vi "PS_Testing.vi"() -> ()   [LabVIEW 2012]
uses:
  BotSpeakSubs/BotspeakSettingsUsed.vi
  SubVIs/LVPresent_Globals.vi
panel:
  out "Button":bool
  out "Light":u8(slide) scale=0.0..255.0
  in  "LED":cluster{"Red":bool, "Green":bool, "Blue":bool}
  # "Test the ProtoSnap\n\nTry pushing the button or reading the light sensor.  You can click on any of the areas to see the program that is running"
  # "Click these to turn on LEDs!"
  # "Move your finger over the sensor to see the bar change!"
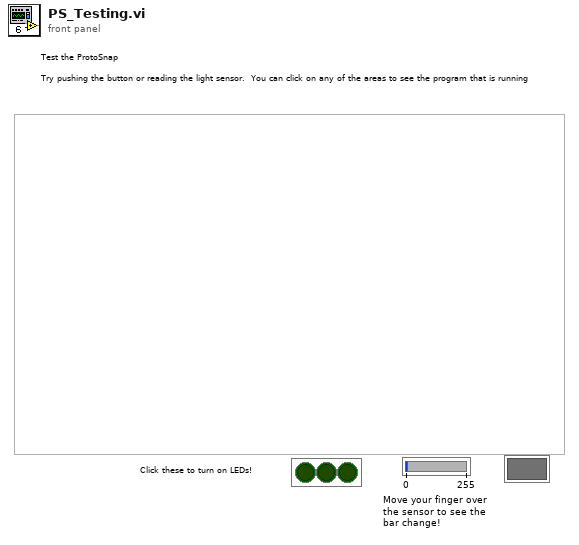
[diagram p1: front panel]
types:
  T1 = typedef "BotSpeak_Control.ctl" = cluster{"Address":string, "Reply EOF":string, "Hardware":string, "Retries":i8, "Timeout":i32}
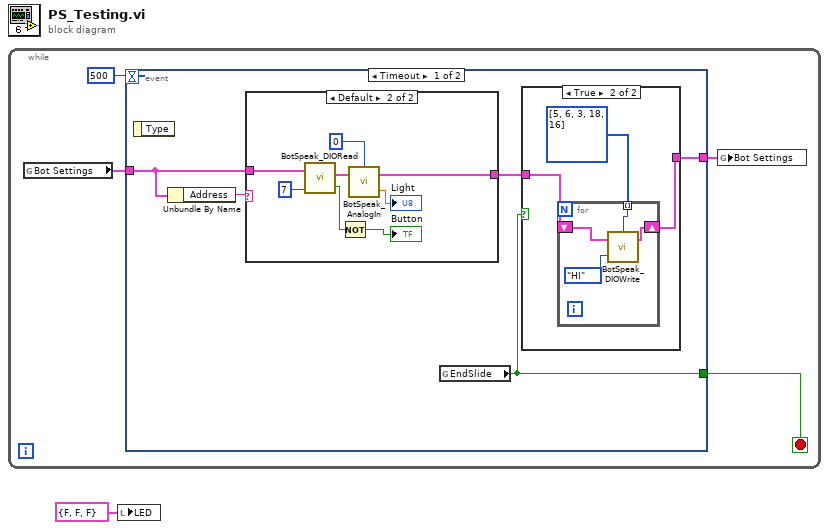
[diagram p0: block diagram]
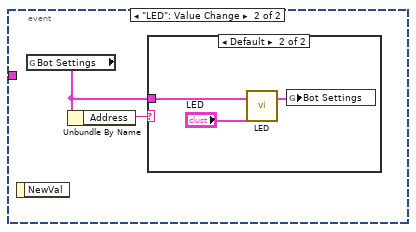
[diagram p4: hidden frame]
diagram:
  n1 = while {
    stop <- w5 stop-if-true
    n2 = global read "BotspeakSettingsUsed.vi" "Bot Settings"() -> (w3:T1)
    n3 = event shown="[0] Timeout" {
      selector: _ -> [_ _]
      dyn-events: _ -> [_ _]
      timeout: 500 -> [_ _]
      tunnel: [w10 _] -> w5
      tunnel: w3 -> [w9 _]
      tunnel: [w6 _] -> w2
      event Timeout {
        n4 = event-data() -> ()  [unwired: 1 in, 1 out]
        n5 = Unbundle By Name(w9) -> ("Address"=w8:string)
        n6 = case shown="Default" w8 {
          tunnel: w9 -> [w19 w21]
          tunnel: [w19 w20] -> w7
          frame "" {
          }
          frame Default {
            n7 = call <userlib>:"BotSpeak_DIORead.vi"("Bot Settings"=w21, "DIO Line"=u32 7) -> ("State"=w24:bool, "Bot Settings out"=w23:T1)  [unwired: 1 in]
            n8 = Not(x=w24) -> (.not. x?=→"Button":bool)
            n9 = call <userlib>:"BotSpeak_AnalogIn.vi"("Bot Settings"=w23, "A/D Channel"=u8 0) -> ("voltage"=→"Light":dbl, "Bot Settings"=w20:T1)  [unwired: 1 in]
          }
        }
        n10 = global read "LVPresent_Globals.vi" "EndSlide"() -> (w10:bool)
        n11 = case shown="True" w10 {
          tunnel: w7 -> [w11 w13]
          tunnel: [w11 w12] -> w6
          frame False {
          }
          frame True {
            n12 = for {
              tunnel: i32[] [5, 6, 3, 18, 16] -> [w18] mode=indexing
              shift-right: [w15] -> w12
              shift-left: w13 -> [w16]
              n13 = call <userlib>:"BotSpeak_DIOWrite.vi"("State"=enum32{"LO", "HI"}."HI", "Bot Settings"=w16, "DIO Line"=w18) -> ("Bot Settings"=w15:T1)  [unwired: 1 out]
            }
          }
        }
      }
      event "LED": Value Change {
        n14 = event-data() -> ()  [unwired: 1 in, 1 out]
        n15 = global read "BotspeakSettingsUsed.vi" "Bot Settings"() -> (w29:T1)
        n16 = Unbundle By Name(w29) -> ("Address"=w28:string)
        n17 = case shown="Default" w28 {
          tunnel: w29 -> [_ w31]
          frame "" {
          }
          frame Default {
            n18 = call "LED.vi"("LED"="LED", "Bot Settings"=w31) -> ("Bot Settings out"=w30:T1)  [unwired: 1 in]
            n19 = global write "BotspeakSettingsUsed.vi" "Bot Settings"(w30) -> ()
          }
        }
      }
    }
    n20 = global write "BotspeakSettingsUsed.vi" "Bot Settings"(w2) -> ()
  }
  n21 = local write "LED"(cluster{"Red":bool, "Green":bool, "Blue":bool} {"Red"=FALSE, "Green"=FALSE, "Blue"=FALSE} ("LED")) -> ()
